vi "SIAM-TML-direkt.vi"(7 "UART: 0..3":u8=1 max=3, 8 "error in (no error)":errorcluster, 11 "TSM":T3={"RS232-axis"=255, "axis"=255, "Command"="", "value"=946.0} {"RS232-axis" format="%0d"}) -> (0 "error out":errorcluster, 3 "Array":T2(array[cluster]) {"command" format="%x" items=["end_no_ticket"=4027514895, "end_ticket"=4027518991, "NoOp"=4026531840, "Read ticks"=4026535936, "Read ticks to var"=4026535938, "Read IP"=4043313152, "Read IP into var"=4043313154, "Set IP from var"=4043309059, "Set IP from var, relative"=4043313155, "branchRel_if_equal"=4043374849, "decrement_branchRel_if_equal"=4043374945, "decrement_branchRel_if_greaterequal"=4043375201, "decrement_branchRel_if_greaterequal_withTicket"=4043379297, "decrement_branchRel_if_smaller"=4043375457, "increment_branchRel_if_smaller"=4043375473, "readVar"=4060090368, "writeVar"=4060086273, "copyVar0_from_var1"=4060086275, "math_addToVariable"=4076863488, "math_addVToVariable"=4076863489, "math_subToVariable"=4076863490, "math_subVToVariable"=4076863491, "math_multToVariable"=4076863492, "math_multvToVariable"=4076863493, "math_divideToVariable"=4076863494, "math_divideVToVariable"=4076863495, "math_modToVariable"=4076863496, "math_modVToVariable"=4076863497, "logic_and"=4093640704, "logic_or"=4093640706, "logic_xor"=4093640708, "bitshift"=4093640712, "I2C-write"=335544337, "I2C-read"=335548433, "Cam-SPI-write"=3254779905, "UART0-VC-Baud-write"=469958673, "UART0-VC-Baud-read"=469962768, "UART0-VC-write"=469762065, "UART0-VC-write-Var"=469762067, "UART0-VC-read-availabe-bytes-to-var"=470355970, "UART0-VC-read-availabe-bytes"=470355984, "UART0-VC-read-skip-bytes"=469831681, "UART0-VC-read"=469766160, "UART0-VC-read-Var"=469766162, "UART1-TSM-Baud-write"=486735889, "UART1-TSM-Baud-read"=486739984, "UART1-TSM-write"=486539281, "UART1-TSM-write-Var"=486539283, "UART1-TSM-read-availabe-bytes-to-var"=487133186, "UART1-TSM-read-availabe-bytes"=487133200, "UART1-TSM-read-skip-bytes"=486604801, "UART1-TSM-read-skip-bytes"=486608897, "UART1-TSM-read"=486543376, "UART1-TSM-read-Var"=486543378, "UART2-Laser-Baud-write"=503513105, "UART2-Baud-read"=503517200, "UART2-write"=503316497, "UART2-write-Var"=503316499, "UART2-read-availabe-bytes-to-var"=503910402, "UART2-read-availabe-bytes"=503910416, "UART2-read-skip-bytes"=503386113, "UART2-read"=503320592, "UART2-read-Var"=503320594, "UART3-Baud-write"=520290321, "UART3-Baud-read"=520294416, "UART3-write"=520093713, "UART3-write-Var"=520093715, "UART3-read-availabe-bytes-to-var"=520687618, "UART3-read-availabe-bytes"=520687632, "UART3-read-skip-bytes"=520163329, "UART3-read"=520097808, "UART3-read-Var"=520097810, "IO-read_bank0"=3489665024, "IO-write_bank0"=3489660929, "IO-read_bank1"=3506442240, "IO-write_bank1"=3506438145, "DA0-0_LED365"=2684354561, "DA0-1_LED385"=2685403137, "DA0-2_LED440"=2686451713, "DA0-3_LED470"=2687500289, "DA0-4_LED510"=2688548865, "DA0-5_LED550"=2689597441, "DA0-6_LED590"=2690646017, "DA0-7_LED640"=2691694593, "DA1-0_LED-R"=2701131777, "DA1-1_LED-G"=2702180353, "DA1-2_LED-B"=2703228929, "DA1-3_LED-AF"=2704277505, "DA1-4"=2705326081, "DA1-5"=2706374657, "DA1-6"=2707423233, "DA1-7"=2708471809, "DA2-Laser0"=2717908993, "DA2-Laser1"=2718957569, "DA2-Laser2"=2720006145, "DA2-Laser3"=2721054721, "DA2-Laser4"=2722103297, "Analog-read_AD0-0"=2818576384, "Analog-read-store_AD0-0"=2818572290, "AF-Register-transfer r/w"=2835349505, "AF-Register-read"=2835353600, "AF-Register-read-to-var"=2835353602, "AF-Transfer-from-var"=2835349507, "IO-delay_bank0"=3489923073, "IO-delay_bank0_fromVar"=3489923075, "read_cam_clock"=3289124864, "store_cam_clock"=3289120770, "read_cam_phase"=3289190400, "store_cam_phase"=3289186306, "store_cam_phase-t"=3289190402, "r_cam1_NHS"=3254980608, "w_cam1_NHS"=3254976513, "r_cam1_NVS"=3255046144, "w_cam1_NVS"=3255042049, "r_cam1_npx"=3255111680, "w_cam1_npx"=3255107585, "r_cam1_npy"=3255177216, "w_cam1_npy"=3255173121, "r_cam1_xhswait"=3255439360, "w_cam1_xhswait"=3255435265, "r_cam1_xvs_wait"=3255504896, "w_cam1_xvs_wait"=3255500801, "r_cam1_framcounter"=3255570432, "r_cam1_line"=3255635968, "r_cam1_xhs-counter"=3255701504, "r_cam2_NHS"=3271757824, "w_cam2_NHS"=3271753729, "r_cam2_NVS"=3271823360, "w_cam2_NVS"=3271819265, "r_cam2_npx"=3271888896, "w_cam2_npx"=3271884801, "r_cam2_npy"=3271954432, "w_cam2_npy"=3271950337, "r_cam2_xvs_wait"=3272282112, "w_cam2_xvs_wait"=3272278017, "r_cam2_framcounter"=3272347648, "r_cam2_line"=3272413184, "r_cam2_xhs-counter"=3272478720, "start TMSI"=102694919, "set_1Galvo"=101712113, "set_x-Galvo"=102760689, "set_y-Galvo"=103809265, "set_z-Fokus"=104857841, "set_1Galvo_position-only"=101711937, "set_x-Galvo_position-only"=102760513, "set_y-Galvo_position-only"=103809089, "set_z-Fokus_position-only"=104857665, "set_x-Galvo_position-only_ticket"=102764609, "set_y-Galvo_position-only_ticket"=103813185, "set_z-Fokus_position-only_ticket"=104861761, "set_1Galvo_relativ-only"=101712001, "set_x-Galvo_relativ-only"=102760577, "set_y-Galvo_relativ-only"=103809153, "set_z-Fokus_relativ-only"=104857729, "set_1Galvo_speed-only"=101711905, "set_x-Galvo_speed-only"=102760481, "set_y-Galvo_speed-only"=103809057, "set_z-Fokus_speed-only"=104857633, "set_1Galvo_acc-only"=101711889, "set_x-Galvo_acc-only"=102760465, "set_y-Galvo_acc-only"=103809041, "set_z-Fokus_acc-only"=104857617, "read_1Galvo_ticket"=101716032, "read_x-Galvo_ticket"=102764608, "read_y-Galvo_ticket"=103813184, "read_z-Focus_ticket"=104861760, "x-Galvo_pos_fromVar"=102760515, "y-Galvo_pos_fromVar"=103809091, "z-Focus_pos_fromVar"=104857667, "Servo0"=67108865, "Servo0-enable"=68091911, "Servo0-disable"=68091919, "Servo1"=68157441, "Servo1-enable"=69140487, "Servo1-disable"=69140495, "Servo2-enable"=70189063, "Servo2"=69206017, "Servo3-enable"=71237639, "Servo3"=70254593, "x-ssi-init"=202309639, "x-ssi-disable"=202309647, "x-ssi-Bits"=201523201, "x-ssi-Read"=201330688, "x-ssi-ReadToVar"=201326594, "x-ssi-ReadToVar-ticket"=201330690, "y-ssi-init"=203358215, "y-ssi-disable"=203358223, "y-ssi-Bits"=202571777, "y-ssi-Read"=202379264, "y-ssi-ReadToVar"=202375170, "y-ssi-ReadToVat-ticket"=202379266]; "P5-ticket" format="%.0x"; "Delay 10µs" format="%.0x"; "P0" format="%.0x"; "P1" format="%.0x"}, 4 "command byte array":u8[](array[numeric])=[6, 0, 16, 118, 1, 3, 178, 66] format="%02x", 5 "expect return":T4(ring))   [LabVIEW 2011]
uses:
  SIAM_command.ctl
panel:
  out "*(type *) &x":u32[](array[numeric]) format="%.0x"
  # "Technosoft default 1\nno used so far! fix1>1D"
  # "reed needs to wait some 10 ms!!!\nexpect at least 1byte: 4F\nstd return data has 9byte, 2-4data,1crc"
  # "cpos=\nupd\nsap 0\ngoto abs\ngoto cal\nTILL_Status=0\n?tpos\n?absposssi\nlsactive=1\nfaultr"
  # "123"
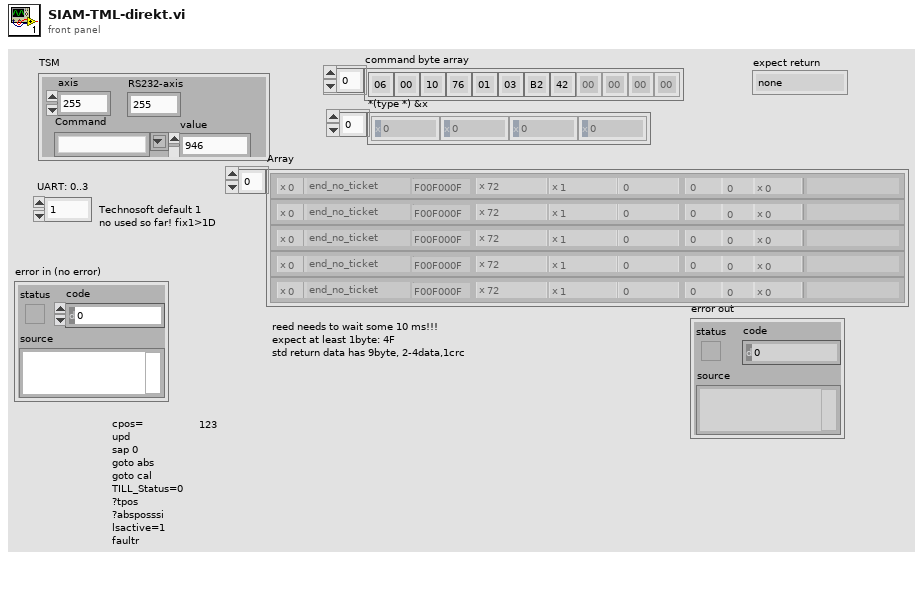
[diagram p1: front panel]
types:
  T1 = typedef "SIAM_command.ctl" = u32
  T2 = cluster{"Delay 10µs":u32, "command":T1, "P0":i32, "P1":i32, "P2":i32, "P3":i32, "P4":i32, "P5-ticket":i32, "comment":string}[]
  T3 = cluster{"RS232-axis":u8, "axis":u8, "Command":string, "value":dbl}
  T4 = enum8{"none", "program32", "program16", "data32", "data16", "eprom32", "eprom16", "somethingelse32", "somethingelse16"}
  T5 = cluster{"Delay 10µs":u32, "command":T1, "P0":i32, "P1":i32, "P2":i32, "P3":i32, "P4":i32, "P5-ticket":i32, string}
  T6 = cluster{"Delay 10µs":u32, "command":T1, "P0":i32, "P1":i32, "P2":i32, "P3":i32, "P4":i32, "P5-ticket":i32, string}[]
  T7 = cluster{"Delay 10µs":u32, "command":T1, "P0":i32, "P1":i32, "P2":i32, "P3":i32, "P4":i32, "P5-ticket":i32, "Comment":string}[]
  T8 = cluster{"Delay 10µs":u32, "command 2":T1, "P0":i32, "P1":i32, "P2":i32, "P3":i32, "P4":i32, "P5-ticket":i32, string}
  T9 = cluster{"Delay 10µs":u32, "command 2":T1, "P0":i32, "P1":i32, "P2":i32, "P3":i32, "P4":i32, "P5-ticket":i32, string}[]
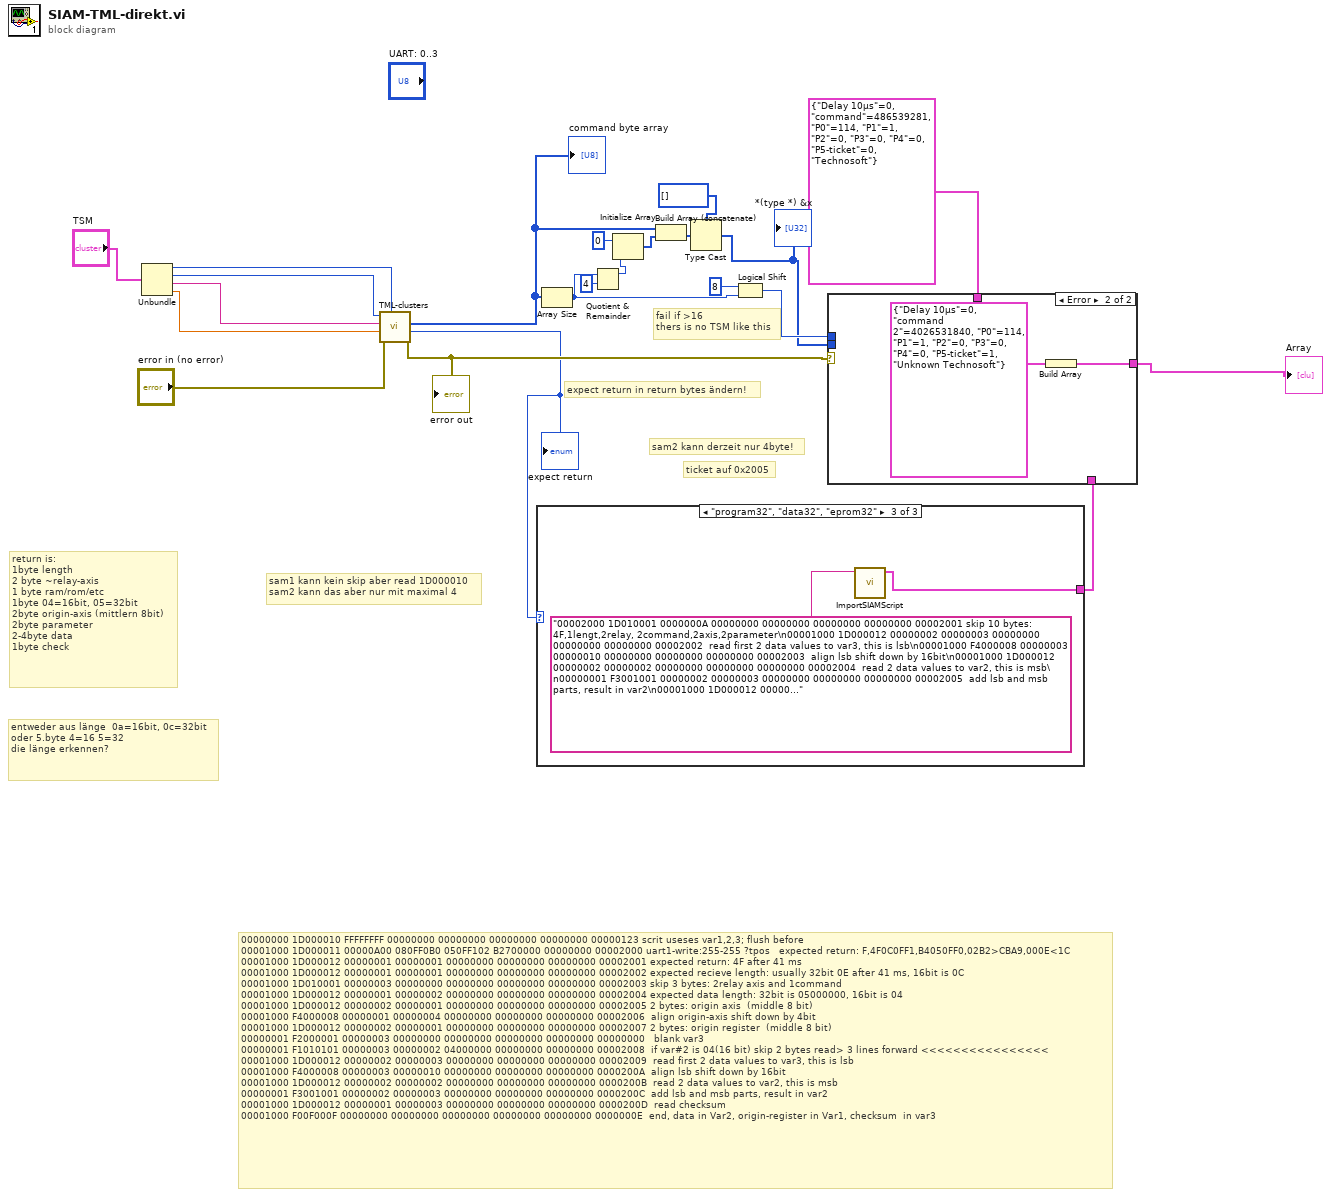
[diagram p0: block diagram]
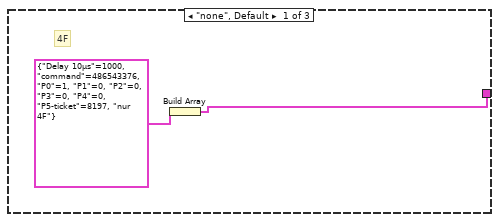
[diagram p2: hidden frame]
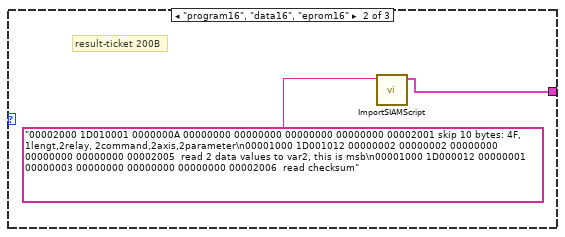
[diagram p3: hidden frame]
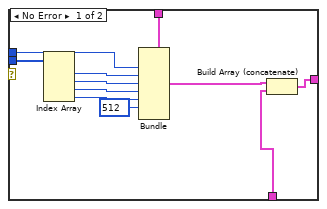
[diagram p4: hidden frame]
diagram:
  # "sam1 kann kein skip aber read 1D000010\nsam2 kann das aber nur mit maximal 4"
  # "ticket auf 0x2005"
  # "00000000 1D000010 FFFFFFFF 00000000 00000000 00000000 00000000 00000123 scrit useses var1,2,3; flush before\n00001000 1D000011 00000A00 080FF0B0 050FF102 B2700000 00000000 00002000 uart1-write:255-255 ?tpos   expected return: F,4F0C0FF1,B4050FF0,02B2>CBA9,000E<1C\n00001000 1D000012 00000001 00000001 00000000 00000000 00000000 00002001 expected return: 4F after 41 ms\n00001000 1D000012 00000001 00000001 00000000 00000000 00000000 00002002 expected recieve length: usually 32bit 0E after 41 ms, 16bit is 0C\n00001000 1D010001 00000003 00000000 00000000 00000000 00000000 00002003 skip 3 bytes: 2relay axis and 1command\n00001000 1D000012 00000001 00000002 00000000 00000000 00000000 00002004 expected data length: 32bit is 05000000, 16bit is 04\n00001000 1D000012 00000002 00000001 00000000 00000000 00000000 00002005 2 bytes: origin axis  (middle 8 bit)\n00001000 F4000008 00000001 00000004 00000000 00000000 00000000 00002006  align origin-axis shift down by 4bit\n00001000 1D000012 00000002 00000001 00000000 00000000 00000000 00002007 2 bytes: origin register  (middle 8 bit)\n00000001 F2000001 00000003 00000000 00000000 00000000 00000000 00000000   blank var3\n00000001 F1010101 00000003 00000002 04000000 00000000 00000000 00002008  if var#2 is 04(16 bit) skip 2 bytes read> 3 lines forward <<<<<<<<<<<<<<<<\n00001000 1D000012 00000002 00000003 00000000 00000000 00000000 00002009  read first 2 data values to var3, this is lsb\n00001000 F4000008 00000003 00000010 00000000 00000000 00000000 0000200A  align lsb shift down by 16bit\n00001000 1D000012 00000002 00000002 00000000 00000000 00000000 0000200B  read 2 data values to var2, this is msb\n00000001 F3001001 00000002 00000003 00000000 00000000 00000000 0000200C  add lsb and msb parts, result in var2\n00001000 1D000012 00000001 00000003 00000000 00000000 00000000 0000200D  read checksum\n00001000 F00F000F 00000000 00000000 00000000 00000000 00000000 0000000E  end, data in Var2, origin-register in Var1, checksum  in var3"
  # "entweder aus länge  0a=16bit, 0c=32bit\noder 5.byte 4=16 5=32\ndie länge erkennen?"
  # "return is:\n1byte length\n2 byte ~relay-axis\n1 byte ram/rom/etc\n1byte 04=16bit, 05=32bit\n2byte origin-axis (mittlern 8bit)\n2byte parameter\n2-4byte data\n1byte check"
  # "expect return in return bytes ändern!"
  # "sam2 kann derzeit nur 4byte!"
  # "fail if >16\nthers is no TSM like this"
  n1 = Unbundle("TSM") -> ("RS232-axis"=w6:u8, "axis"=w7:u8, "Command"=w5:string, "value"=w4:dbl)
  n2 = call "TML-clusters.vi"("RS232-axis"=w6, "error in (no error)"="error in (no error)", "value"=w4, "command"=w5, "axis"=w7) -> ("error out"=w15:errorcluster, "expect return"=w3:T4, "command byte array"=w21:u8[])  [unwired: 4 in]
  "command byte array" <- w21
  "expect return" <- w3
  "error out" <- w15
  n3 = case shown="\"program32\", \"data32\", \"eprom32\"" w3 {
    tunnel: [w23 w26 w28] -> w2
    frame "none", Default {
      # "4F"
      n4 = Build Array(T5 {"Delay 10µs"=1000, "command"=486543376, "P0"=1, "P1"=0, "P2"=0, "P3"=0, "P4"=0, "P5-ticket"=8197, "nur 4F"} ("SAM-command 2")) -> (w23:T6)
    }
    frame "program16", "data16", "eprom16" {
      # "result-ticket 200B"
      n5 = call "ImportSIAMScript.vi"("String"="00002000 1D010001 0000000A 00000000 00000000 00000000 00000000 00002001 skip 10 bytes: 4F, 1lengt,2relay, 2command,2axis,2parameter\n00001000 1D001012 00000002 00000002 00000000 00000000 00000000 00002005  read 2 data values to var2, this is msb\n00001000 1D000012 00000001 00000003 00000000 00000000 00000000 00002006  read checksum") -> ("Script"=w26:T7)  [unwired: 9 in, 1 out]
    }
    frame "program32", "data32", "eprom32" {
      n6 = call "ImportSIAMScript.vi"("String"="00002000 1D010001 0000000A 00000000 00000000 00000000 00000000 00002001 skip 10 bytes: 4F,1lengt,2relay, 2command,2axis,2parameter\n00001000 1D000012 00000002 00000003 00000000 00000000 00000000 00002002  read first 2 data values to var3, this is lsb\n00001000 F4000008 00000003 00000010 00000000 00000000 00000000 00002003  align lsb shift down by 16bit\n00001000 1D000012 00000002 00000002 00000000 00000000 00000000 00002004  read 2 data values to var2, this is msb\n00000001 F3001001 00000002 00000003 00000000 00000000 00000000 00002005  add lsb and msb parts, result in var2\n00001000 1D000012 00000001 00000003 00000000 00000000 00000000 00002006  read checksum") -> ("Script"=w28:T7)  [unwired: 9 in, 1 out]
    }
  }
  n7 = Array Size(array=w21) -> (size(s)=w11:i32)
  n8 = Quotient & Remainder(x=w11, y=4) -> (x-y*floor(x/y)=w9:i32)  [unwired: 1 out]
  n9 = Initialize Array(u8 0, w9) -> (w12:u8[])
  n10 = Build Array (concatenate)(w21, w12) -> (w14:u8[])
  n11 = Type Cast(type=u32[] [], x=w14) -> (*(type *) &x=w16:u32[])
  "*(type *) &x" <- w16
  n12 = Logical Shift(y=i8 8, x=w11) -> (x << y=w17:i32)
  n13 = case shown="Error" w15 {
    tunnel: T5 {"Delay 10µs"=0, "command"=486539281, "P0"=114, "P1"=1, "P2"=0, "P3"=0, "P4"=0, "P5-ticket"=0, "Technosoft"} ("SAM-command 2") -> [w39 _]
    tunnel: w17 -> [w38 _]
    tunnel: w16 -> [w37 _]
    tunnel: [w29 w40] -> w1
    tunnel: w2 -> [w30 _]
    frame No Error {
      n14 = Index Array(array=w37) -> (element #1=w36:u32, element #2=w35:u32, element #3=w34:u32, element #4=w33:u32)  [unwired: 4 in]
      n15 = Bundle(cluster=w39, "P0"=w38, "P1"=w36, "P2"=w35, "P3"=w34, "P4"=w33, "P5-ticket"=512) -> (w31:T5)  [unwired: 3 in]
      n16 = Build Array (concatenate)(w31, w30) -> (w29:T7)
    }
    frame Error {
      n17 = Build Array(T8 {"Delay 10µs"=0, "command 2"=4026531840, "P0"=114, "P1"=1, "P2"=0, "P3"=0, "P4"=0, "P5-ticket"=1, "Unknown Technosoft"} ("SAM-command 2")) -> (w40:T9)
    }
  }
  "Array" <- w1
